vi "LabelBinarizer.vi"(8 "error in (no error)":errorcluster caption="entrée d'erreur (pas d'erreur)", 11 "LabelBinarizer":T1={"neg_label"=0, "pos_label"=1, "sparse_output"=FALSE}) -> (0 "error out":errorcluster, 3 "LabelBinarizer.lvclass":refnum<class "LabelBinarizer.lvclass">)   [LabVIEW 2020]
doc: "Binarize labels in a one-vs-all fashion\n\nSeveral regression and binary classification algorithms are available in scikit-learn. A simple way to extend these algorithms to the multi-class classification case is to use the so-called one-vs-all scheme.\n\nAt learning time, this simply consists in learning one regressor or binary classifier per class. In doing so, one needs to convert multi-class labels to binary labels (belong or does not belong to the class). LabelBinarizer makes this process easy with the transform method.\n\nAt prediction time, one assigns the class for which the corresponding model gave the greatest confidence. LabelBinarizer makes this easy with the inverse_transform method.\n\n\nParameters : \n\n- neg_label : int (default: 0)\nValue with which negative labels must be encoded.\n\n- pos_label : int (default: 1)\nValue with which positive labels must be encoded.\n\n- sparse_output : boolean (default: False)\nTrue if the returned array from transform is desired to be in sparse CSR format.\n\n\nMethods : \n\n\n- Fit : Fit label binarizer\n\nParameters : y : array of shape [n_samples,] or [n_samples, n_classes]\n Target values. The 2-d matrix should only contain 0 and 1, represents multilabel classification.\n\n\n- Fit Transform : Fit label binarizer and transform multi-class labels to binary labels. The output of transform is sometimes referred to as the 1-of-K coding scheme.\n\nParameters : y : array or sparse matrix of shape [n_samples,] or [n_samples, n_classes]\n Target values. The 2-d matrix should only contain 0 and 1, represents multilabel classification. Sparse matrix can be CSR, CSC, COO, DOK, or LIL.\n\nReturns : Y : array or CSR matrix of shape [n_samples, n_classes]\n Shape will be [n_samples, 1] for binary problems.\n\n\n- Transform : Transform multi-class labels to binary labels. The output of transform is sometimes referred to by some authors as the 1-of-K coding scheme.\n\nParameters : y : array or sparse matrix of shape [n_samples,] or [n_samples, n_classes]\n Target values. The 2-d matrix should only contain 0 and 1, represents multilabel classification. Sparse matrix can be CSR, CSC, COO, DOK, or LIL.\n\nReturns : Y : numpy array or CSR matrix of shape [n_samples, n_classes]\n Shape will be [n_samples, 1] for binary problems."
uses:
  LabelBinarizer.lvclass
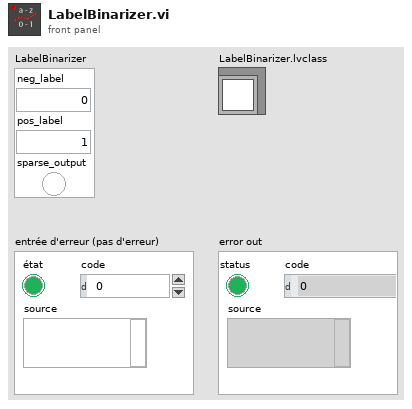
[diagram p1: front panel]
types:
  T1 = cluster{"neg_label":i32, "pos_label":i32, "sparse_output":bool}
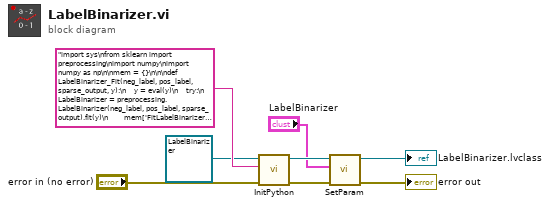
[diagram p0: block diagram]
diagram:
  n1 = call-dynamic "InitPython.vi"("error in (no error)"="error in (no error)", "Python Instruction"="import sys\nfrom sklearn import preprocessing\nimport numpy\nimport numpy as np\n\nmem = {}\n\n\ndef LabelBinarizer_Fit(neg_label, pos_label, sparse_output, y):\n    y = eval(y)\n    try:\n        LabelBinarizer = preprocessing.LabelBinarizer(neg_label, pos_label, sparse_output).fit(y)\n        mem['FitLabelBinarizer'] = LabelBinarizer\n        return str('OK')\n    except:\n        erreur = sys.exc_info()\n        typerr = u\"%s\" % (erreur[0])\n        typerr = typerr[typerr.find(\"'\")+1:typerr.rfind(\"'\")]\n        msgerr = u\"%s\" % (erreur[1])\n        message = str('/!\\\\ {0} : {1}'. format(typerr,msgerr))\n        return message \n    \ndef LabelBinarizer_FitTransform(neg_label, pos_label, sparse_output, y):\n    y = eval(y)\n    try:\n        LabelBinarizer = preprocessing.LabelBinarizer(neg_label, pos_label, sparse_output).fit_transform(y)\n        dtype = type(LabelBinarizer)\n        if dtype == numpy.ndarray:\n            LabelBinarizer = LabelBinarizer.tolist()\n            return str(LabelBinarizer) \n        else:\n            Mat = LabelBinarizer.tocoo()\n            return str(list(zip(Mat.row, Mat.col, Mat.data)))\n    except:\n        erreur = sys.exc_info()\n        typerr = u\"%s\" % (erreur[0])\n        typerr = typerr[typerr.find(\"'\")+1:typerr.rfind(\"'\")]\n        msgerr = u\"%s\" % (erreur[1])\n        message = str('/!\\\\ {0} : {1}'. format(typerr,msgerr))\n        return message \n\ndef LabelBinarizer_Transform(neg_label, pos_label, sparse_output, y): #sparse_output renvoie une matrice creuse si Vrai\n    y = eval(y)\n    try:\n        LabelBinarizer = mem['FitLabelBinarizer'].transform(y)\n        dtype = type(LabelBinarizer)\n        if dtype == numpy.ndarray:\n            LabelBinarizer = LabelBinarizer.tolist()\n            return str(LabelBinarizer) \n        else:\n            Mat = LabelBinarizer.tocoo()\n            return str(list(zip(Mat.row, Mat.col, Mat.data)))\n    except:\n        erreur = sys.exc_info()\n        typerr = u\"%s\" % (erreur[0])\n        typerr = typerr[typerr.find(\"'\")+1:typerr.rfind(\"'\")]\n        msgerr = u\"%s\" % (erreur[1])\n        message = str('/!\\\\ {0} : {1}'. format(typerr,msgerr))\n        return message", "Scikit-learn en entrée"=refnum<class "LabelBinarizer.lvclass"> refnum ("LabelBinarizer.lvclass")) -> ("error out"=w3:errorcluster, "Scikit-learn en sortie"=w5:refnum<class "LabelBinarizer.lvclass">)  [unwired: 7 in]
  n2 = call-dynamic "SetParam.vi"("error in (no error)"=w3, "LabelBinarizer"="LabelBinarizer", "LabelBinarizer.lvclass"=w5) -> ("error out"=→"error out":errorcluster, "LabelBinarizer.lvclass"=→"LabelBinarizer.lvclass":refnum<class "LabelBinarizer.lvclass">)  [unwired: 7 in]
